vi "AKD Set Drive Disable.vi"(0 "connection ID":refnum<k5>, 11 "error in":errorcluster) -> (4 "TCP Refnum":refnum<k5>, 15 "error out":errorcluster)   [LabVIEW 2024]
uses:
  MODBUS/NI Modbus.llb/MB Ethernet Master Query Write Multiple Registers (poly).vi
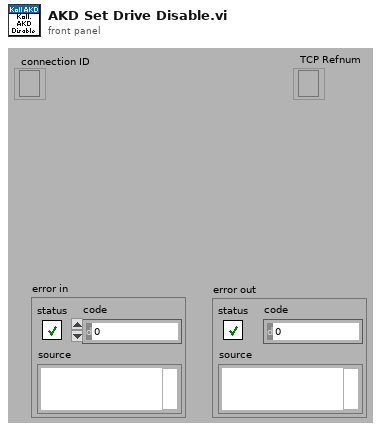
[diagram p1: front panel]
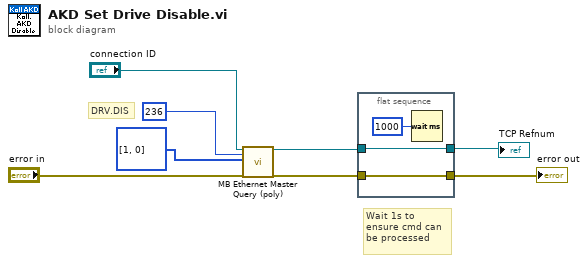
[diagram p0: block diagram]
diagram:
  # "Wait 1s to \nensure cmd can\nbe processed"
  # "DRV.DIS"
  n1 = call-poly "MB Ethernet Master Query (poly).vi"("TCP Connection Refnum in"="connection ID", "Starting Address"=u16 236, "Registers"=u16[] [1, 0], "error in"="error in") -> ("TCP Connection Refnum (dup)"=w4:refnum<k5>, "error out"=w1:errorcluster)  [unwired: 13 in, 1 out]
  n2 = flat-sequence {
    tunnel: [w10] -> w3
    tunnel: w4 -> [w10]
    tunnel: w1 -> [w9]
    tunnel: [w9] -> w2
    frame #0 {
      n3 = Wait (ms)(milliseconds to wait=u32 1000) -> ()  [unwired: 1 out]
    }
  }
  "error out" <- w2
  "TCP Refnum" <- w3
